vi "Benchmark Creation.vi"(8 "error in (no error)":errorcluster, 11 "CIFCorePlugin in":refnum<class "CIFCorePlugin.lvclass">) -> (0 "error out":errorcluster, 3 "CIFCorePlugin out":refnum<class "CIFCorePlugin.lvclass">)   [LabVIEW 2021, in "CIFCorePlugin.lvclass"]
uses:
  CIFCorePlugin.lvclass
  CIFCorePlugin.lvclass/CIFCorePlugin.ctl
  Accessors/Timestamps/Read Creation TS.vi
  Accessors/Get Time.vi
  CIFUtilities/CIFClocks/SubVIs/Add Error.vi
  CIFUtilities/CIFClocks/Core/Get Time.vi
  CIFUtilities/CIFClocks/Time Conversion/LabVIEW Time to UTC Time.vi
  CIFCoreCommon/CIFCoreCommon.lvlib
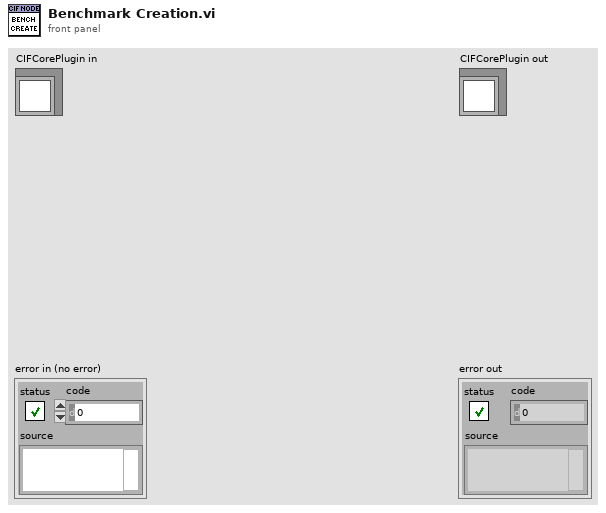
[diagram p1: front panel]
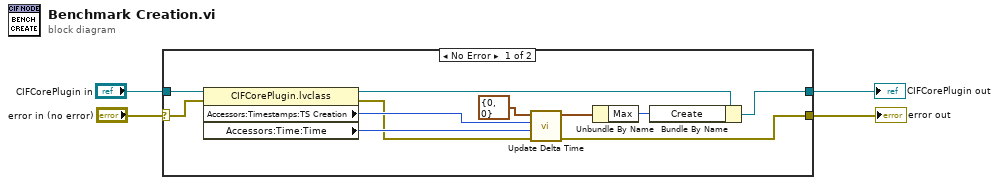
[diagram p0: block diagram]
diagram:
  n1 = case shown="No Error" "error in (no error)" {
    selector: "error in (no error)" -> [w7 w17]
    tunnel: [w11 w17] -> w1
    tunnel: [w12 w16] -> w2
    tunnel: "CIFCorePlugin in" -> [w10 w16]
    frame No Error {
      n2 = property class="CIFCorePlugin.lvclass"(reference=w10, error in=w7) -> (reference out=w9:refnum<class "CIFCorePlugin.lvclass">, error out=w5:errorcluster, "Accessors:Timestamps:TS Creation"=w8:u64, "Accessors:Time:Time"=w6:u64)
      n3 = call "Update Delta Time.vi"("error in (no error)"=w5, "T2"=w6, "T1"=w8, "Timing in"=cluster{"Max":i32, "Min":i32} {"Max"=0, "Min"=0}) -> ("error out"=w11:errorcluster, "Timing out"=w14:cluster{"Max":i32, "Min":i32})  [unwired: 6 in]
      n4 = Unbundle By Name(w14) -> ("Max"=w13:i32)
      n5 = Bundle By Name(cluster=w9, "Create"=w13) -> (w12:refnum<class "CIFCorePlugin.lvclass">)
    }
    frame Error {
    }
  }
  "error out" <- w1
  "CIFCorePlugin out" <- w2
